vi "baustein_einzug.vi"(8 "error in (no error)":errorcluster caption="Fehler (Eingang, kein Fehler)", 11 "Device ID":T1(ring)) -> (0 "error out":errorcluster caption="Fehler (Ausgang)", 3 "Device ID Out":T1(ring))   [LabVIEW 2010]
uses:
  globale Variable 1.vi
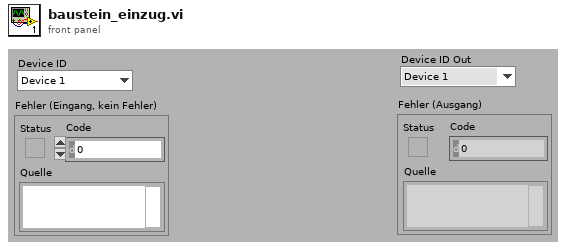
[diagram p1: front panel]
types:
  T1 = enum16{"Device 1", "Device 2", "Device 3", "Device 4", "Device 5", "Device 6", "Device 7", "Device 8"}
  T2 = enum8{"Power 1", "Power 2", "Power 3", "Power 4", "Power 5", "Power 6", "Power 7", "Power 8"}
  T3 = enum8{"Output 1 (O1)", "Output 2 (O2)", "Output 3 (O3)", "Output 4 (O4)", "Output 5 (O5)", "Output 6 (O6)", "Output 7 (O7)", "Output 8 (O8)"}
  T4 = enum8{"Robo Interface", "Extension 1", "Extension 2", "Extension 3"}
  T5 = enum8{"Goes High", "Goes Low", "Goes High or Low"}
  T6 = enum8{"Input 1 (I1)", "Input 2 (I2)", "Input 3 (I3)", "Input 4 (I4)", "Input 5 (I5)", "Input 6 (I6)", "Input 7 (I7)", "Input 8 (I8)"}
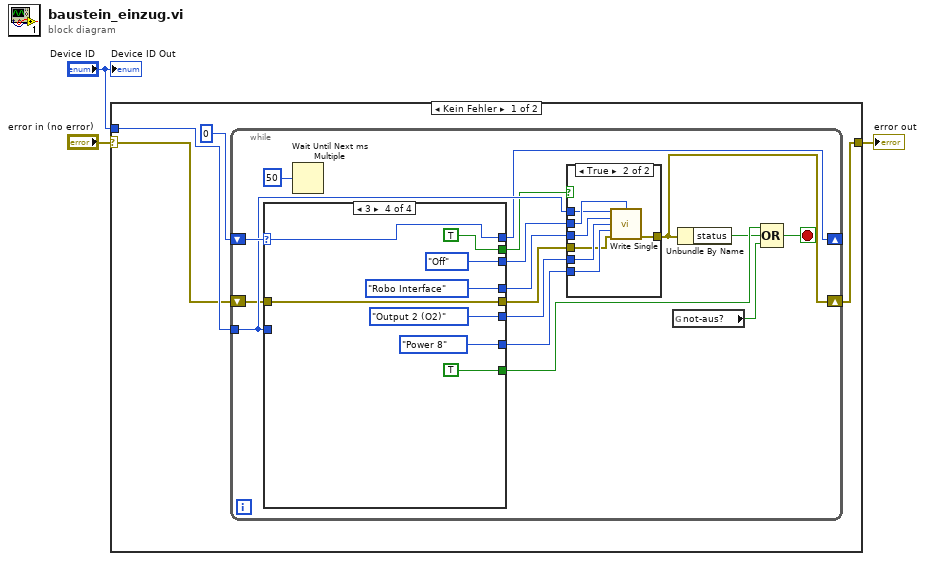
[diagram p0: block diagram]
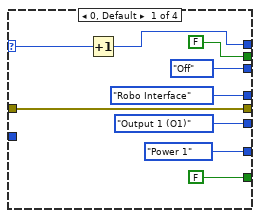
[diagram p2: hidden frame]
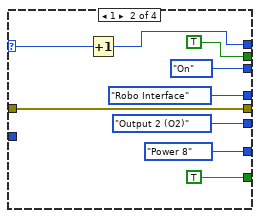
[diagram p3: hidden frame]
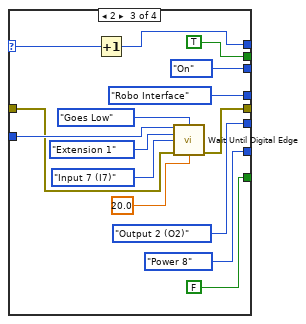
[diagram p4: hidden frame]
diagram:
  n1 = case shown="Kein Fehler" "error in (no error)" {
    selector: "error in (no error)" -> [w6 w73]
    tunnel: [w5 w73] -> w2
    tunnel: "Device ID" -> [w7 _]
    frame No Error {
      n2 = while {
        tunnel: w7 -> [w21]
        shift-right: [w11] -> w5
        shift-left: w6 -> [w18]
        shift-right: [w20] -> _
        shift-left: 0 -> [w22]
        stop <- w10 stop-if-true
        n3 = case shown="3" w22 {
          selector: w22 -> [w32 w41 w56 w57]
          tunnel: w21 -> [_ _ w45 _]
          tunnel: [w31 w40 w55 w57] -> w20
          tunnel: [FALSE TRUE TRUE TRUE] -> w16
          tunnel: [w29 w37 w43 w58] -> w19
          tunnel: w18 -> [w29 w37 w44 w58]
          tunnel: [FALSE TRUE FALSE TRUE] -> w17
          tunnel: [T2."Power 1" ("Output_PWM") T2."Power 8" ("Output_PWM") T2."Power 8" ("Output_PWM") T2."Power 8" ("Output_PWM")] -> w15
          tunnel: [T3."Output 1 (O1)" ("Single_Output") T3."Output 2 (O2)" ("Single_Output") T3."Output 2 (O2)" ("Single_Output") T3."Output 2 (O2)" ("Single_Output")] -> w14
          tunnel: [T4."Robo Interface" ("Module") T4."Robo Interface" ("Module") T4."Robo Interface" ("Module") T4."Robo Interface" ("Module")] -> w13
          tunnel: [enum8{"Off", "On"}."Off" ("Output_Action") enum8{"Off", "On"}."On" ("Output_Action") enum8{"Off", "On"}."On" ("Output_Action") enum8{"Off", "On"}."Off" ("Output_Action")] -> w12
          frame 0, Default {
            n4 = Increment(x=w32) -> (x+1=w31:i32)
          }
          frame 1 {
            n5 = Increment(x=w41) -> (x+1=w40:i32)
          }
          frame 2 {
            n6 = Increment(x=w56) -> (x+1=w55:i32)
            n7 = call "Wait Until Digital Edge.vi"("Device ID"=w45, "Wait Until"=T5."Goes Low", "Module"=T4."Extension 1", "Digital_Input"=T6."Input 7 (I7)", "error in"=w44, "Time Out (10)"=20.0) -> ("error out"=w43:errorcluster)  [unwired: 9 out]
          }
          frame 3 {
          }
        }
        n8 = Wait Until Next ms Multiple(millisecond multiple=50) -> ()  [unwired: 1 out]
        n9 = case shown="TRUE" w16 {
          tunnel: w14 -> [_ w72]
          tunnel: w13 -> [_ w71]
          tunnel: w12 -> [_ w70]
          tunnel: w15 -> [_ w69]
          tunnel: w21 -> [_ w68]
          tunnel: w19 -> [w65 w67]
          tunnel: [w65 w66] -> w11
          frame False {
          }
          frame True {
            n10 = call "Write Single.vi"("Device ID"=w68, "Output_Action"=w70, "Module"=w71, "Single_Output"=w72, "Output_PWM"=w69, "error in"=w67) -> ("error out"=w66:errorcluster)  [unwired: 9 out]
          }
        }
        n11 = global read "globale Variable 1.vi" "not-aus?"() -> (w8:bool)
        n12 = Unbundle By Name(w11) -> ("status"=w9:bool)
        n13 = Compound Arithmetic op=OR(w17, w9, w8) -> (w10:bool)
      }
    }
    frame Error {
    }
  }
  "error out" <- w2
  "Device ID Out" <- "Device ID"
